vi "Group Spectrum Lines.vi"(0 "spectra":T2(array[cluster]), 9 "system info in":refnum<class "EP System Info.lvclass">, 11 "error in (no error)":errorcluster) -> (4 "harmonic groups complex spectra":cluster{"f0":dbl, "df":dbl, "vectors":cdb[]}[](array[cluster]), 6 "interharmonic groups complex spectra":cluster{"f0":dbl, "df":dbl, "vectors":cdb[]}[](array[cluster]), 10 "system info out":refnum<class "EP System Info.lvclass">, 15 "error out":errorcluster)   [LabVIEW 2014, in "NI_EP_Power Quality.lvlib"]
doc: "Groups 10/12-cycle spectra to harmonic and interharmonic spectra according to IEC 61000-4-7:2009. Use the Complex To Polar function to convert the results of this VI to magnitude and phase spectra. Use the Complex To Re/Im function to convert the results of this VI to real and imaginary spectra.\n\nThis VI supports measuring single-line and multiple-line systems."
uses:
  <vilib>/addons/Electrical Power/PQ/NI_EP_Power Quality.lvlib
  <vilib>/addons/Electrical Power/PQ/Common/Controls/ep_AI Data Channel.ctl
  <vilib>/addons/Electrical Power/PQ/Common/Classes/System Info/EP System Info.lvclass
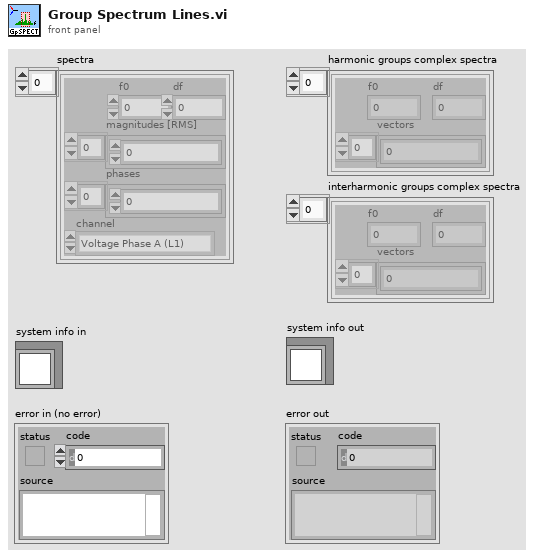
[diagram p1: front panel]
types:
  T1 = typedef "NI_EP_Power Quality.lvlib/ep_AI Data Channel.ctl" = enum16{"Voltage Phase A (L1)", "Voltage Phase B (L2)", "Voltage Phase C (L3)", "Voltage Phase N (Neutral)", "Current Phase A (L1)", "Current Phase B (L2)", "Current Phase C (L3)", "Current Phase N (Neutral)"}
  T2 = cluster{"f0":dbl, "df":dbl, "magnitudes [RMS]":dbl[], "phases":dbl[], "channel":T1}[]
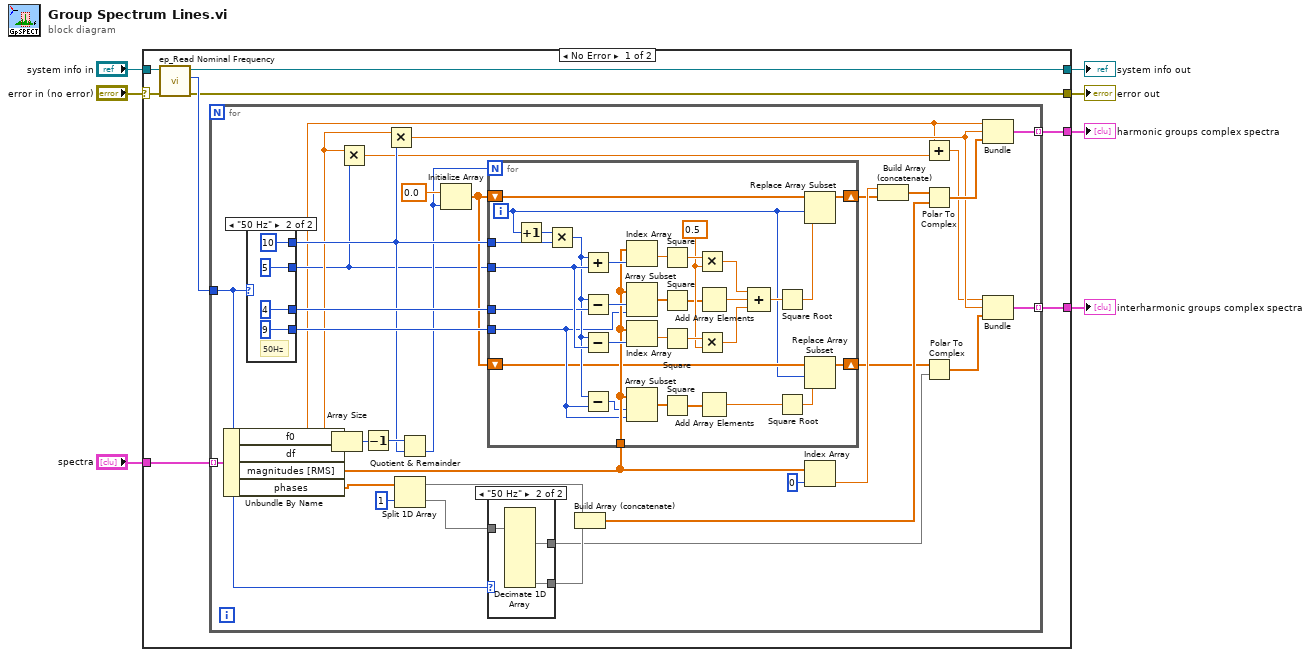
[diagram p0: block diagram]
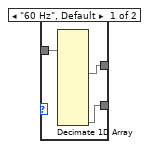
[diagram p2: hidden frame]
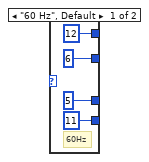
[diagram p3: hidden frame]
diagram:
  n1 = case shown="No Error" "error in (no error)" {
    selector: "error in (no error)" -> [w12 w96]
    tunnel: "spectra" -> [w14 _]
    tunnel: "system info in" -> [w13 w95]
    tunnel: [w11 w96] -> w2
    tunnel: [w10 w95] -> w3
    tunnel: [w9 _] -> w4
    tunnel: [w8 _] -> w1
    frame No Error {
      n2 = call <vilib>:"ep_Read Nominal Frequency.vi"("error in (no error)"=w12, "system info in"=w13) -> ("error out"=w11:errorcluster, "nominal frequency"=w15:enum16{"50 Hz", "60 Hz"}, "system info out"=w10:refnum<class "EP System Info.lvclass">)  [unwired: 6 in, 1 out]
      n3 = for {
        tunnel: w15 -> [w40]
        tunnel: w14 -> [w44] mode=indexing
        tunnel: [w43] -> w9 mode=indexing
        tunnel: [w23] -> w8 mode=indexing
        n4 = Unbundle By Name(w44) -> ("f0"=w18:dbl, "df"=w20:dbl, "magnitudes [RMS]"=w28:dbl[], "phases"=w27:dbl[])
        n5 = case shown="\"50 Hz\"" w40 {
          tunnel: [12 ("x") 10 ("x")] -> w30
          tunnel: [5 ("y") 4 ("y")] -> w46
          tunnel: [11 ("Array Length") 9 ("Array Length")] -> w45
          tunnel: [6 ("y") 5 ("y")] -> w19
          frame "60 Hz", Default {
            # "60Hz"
          }
          frame "50 Hz" {
            # "50Hz"
          }
        }
        n6 = Array Size(array=w28) -> (size(s)=w32:i32)
        n7 = Multiply(x=w20, y=w19) -> (x*y=w17:dbl)
        n8 = Decrement(x=w32) -> (x-1=w31:i32)
        n9 = Multiply(x=w20, y=w30) -> (x*y=w24:dbl)
        n10 = Split 1D Array(array=w27, index=1) -> (first subarray=w36:dbl[], second subarray=w37:dbl[])
        n11 = Quotient & Remainder(x=w31, y=w30) -> (floor(x/y)=w29:i32)  [unwired: 1 out]
        n12 = Initialize Array(0.0 ("Element Data"), w29) -> (w22:dbl[])
        n13 = for {
          N: w29 -> [_]
          shift-right: [w93] -> w34
          shift-left: w22 -> [w94]
          tunnel: w28 -> [w71]
          tunnel: w30 -> [w90]
          tunnel: w19 -> [w92]
          tunnel: w46 -> [w91]
          tunnel: w45 -> [w67]
          shift-right: [w65] -> w21
          shift-left: w22 -> [w66]
          i -> [w63]
          w80 = 0.5 ("y")
          n14 = Increment(x=w63) -> (x+1=w74:i32)
          n15 = Multiply(x=w74, y=w90) -> (x*y=w69:i32)
          n16 = Add(x=w69, y=w92) -> (x+y=w84:i32)
          n17 = Subtract(x=w69, y=w91) -> (x-y=w85:i32)
          n18 = Subtract(x=w69, y=w92) -> (x-y=w86:i32)
          n19 = Subtract(x=w69, y=w67) -> (x-y=w68:i32)
          n20 = Index Array(array=w71, index=w84) -> (element=w89:dbl)
          n21 = Array Subset(array=w71, index=w85, length=w67) -> (w87:dbl[])
          n22 = Index Array(array=w71, index=w86) -> (element=w88:dbl)
          n23 = Array Subset(array=w71, index=w68, length=w67) -> (w72:dbl[])
          n24 = Square(x=w89) -> (x^2=w82:dbl)
          n25 = Square(x=w87) -> (x^2=w79:dbl[])
          n26 = Square(x=w88) -> (x^2=w81:dbl)
          n27 = Square(x=w72) -> (x^2=w73:dbl[])
          n28 = Multiply(x=w82, y=w80) -> (x*y=w77:dbl)
          n29 = Multiply(x=w81, y=w80) -> (x*y=w76:dbl)
          n30 = Add Array Elements(numeric array=w79) -> (sum=w78:dbl)
          n31 = Add Array Elements(numeric array=w73) -> (sum=w70:dbl)
          n32 = Compound Arithmetic op=ADD(w77, w78, w76) -> (w75:dbl)
          n33 = Square Root(x=w75) -> (sqrt(x)=w83:dbl)
          n34 = Square Root(x=w70) -> (sqrt(x)=w64:dbl)
          n35 = Replace Array Subset(array=w94, new element=w83, index=w63) -> (w93:dbl[])
          n36 = Replace Array Subset(array=w66, new element=w64, index=w63) -> (w65:dbl[])
        }
        n37 = case shown="\"50 Hz\"" w40 {
          tunnel: w37 -> [w51 w54]
          tunnel: [w50 w53] -> w39
          tunnel: [w49 w52] -> w25
          frame "60 Hz", Default {
            n38 = Decimate 1D Array(w51) -> (w49:dbl[], w50:dbl[])  [unwired: 10 out]
          }
          frame "50 Hz" {
            n39 = Decimate 1D Array(w54) -> (w52:dbl[], w53:dbl[])  [unwired: 8 out]
          }
        }
        n40 = Build Array (concatenate)(w36, w39) -> (w42:dbl[])
        n41 = Index Array(array=w28, index=0 ("Index")) -> (element=w35:dbl)
        n42 = Build Array (concatenate)(w35, w34) -> (w33:dbl[])
        n43 = Add(x=w18, y=w17) -> (x+y=w16:dbl)
        n44 = Polar To Complex(1:w42, 2:w33) -> (0:w41:cdb[])
        n45 = Polar To Complex(1:w25, 2:w21) -> (0:w26:cdb[])
        n46 = Bundle("f0"=w18, w24, w41) -> (w43:cluster{"f0":dbl, dbl, cdb[]})  [unwired: 1 in]
        n47 = Bundle(w16, w24, w26) -> (w23:cluster{dbl, dbl, cdb[]})  [unwired: 1 in]
      }
    }
    frame Error {
    }
  }
  "error out" <- w2
  "harmonic groups complex spectra" <- w4
  "system info out" <- w3
  "interharmonic groups complex spectra" <- w1
